vi "Wrapper_getSpectrum.vi"(2 "Index":i32, 3 "Wrapper":u32) -> (0 "Length":i32, 1 "Spectrum Values":dbl[](array[numeric]))   [LabVIEW 2017]
uses:
  common32.dll
  OmniDriver32.dll
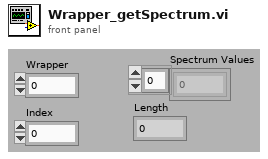
[diagram p1: front panel]
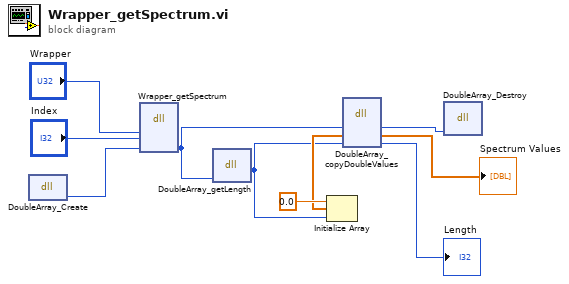
[diagram p0: block diagram]
diagram:
  n1 = dll-call lib="common32.dll" fn="DoubleArray_Create" label="DoubleArray.Create"() -> ("return type"=w8:u32)  [unwired: 3 in, 2 out]
  n2 = dll-call lib="OmniDriver32.dll" fn="Wrapper_getSpectrum" label="Wrapper.getSpectrum"("Wrapper"="Wrapper", "Index"="Index", "DoubbleArray"=w8) -> ("DoubbleArray"=w4:u32)  [unwired: 5 in, 3 out]
  n3 = dll-call lib="common32.dll" fn="DoubleArray_getLength" label="DoubleArray.getLength"("DoubbleArray"=w4) -> ("return type"=w5:i32)  [unwired: 4 in, 2 out]
  n4 = Initialize Array(0.0 ("element"), w5) -> (w6:dbl[])
  n5 = dll-call lib="common32.dll" fn="DoubleArray_copyDoubleValues" label="DoubleArray.copyDoubleValues"("DoubbleArray"=w4, "Values"=w6, "Length"=w5) -> ("DoubbleArray"=w1:u32, "Values"=→"Spectrum Values":dbl[], "Length"=→"Length":i32)  [unwired: 3 in, 3 out]
  n6 = dll-call lib="common32.dll" fn="DoubleArray_Destroy" label="DoubleArray.Destroy"("DoubleArray"=w1) -> ()  [unwired: 4 in, 3 out]
